vi "Reporte_Word.vi"() -> ()   [LabVIEW 2016]
uses:
  <vilib>/addons/_office/_exclsub.llb/font.ctl
  <vilib>/addons/_office/word.llb/Word Easy Table (num).vi
  <vilib>/Utility/NIReport.llb/Append Image to Report (path wrap).vi
  <vilib>/printing/ReportDocExtensions.llb/Append Front Panel Image to Report (path).vi
  <vilib>/printing/ReportDocExtensions.llb/Append VI Block Diagram to Report (path).vi
  <vilib>/Utility/NIReport.llb/NI_report.lvclass
  <vilib>/addons/_office/NI_ReportGenerationToolkit.lvlib
  <vilib>/Utility/NIReport.llb/NI_ReportGenerationCore.lvlib
panel:
  in  "VI":path
  in  "File Path Control":path
  out "Gauge":dbl(knob) scale=0.0..10.0
  in  "path or URL of image":path
  in  "Array":dbl[][](array[numeric])
  in  "String 2":string
  in  "String":string
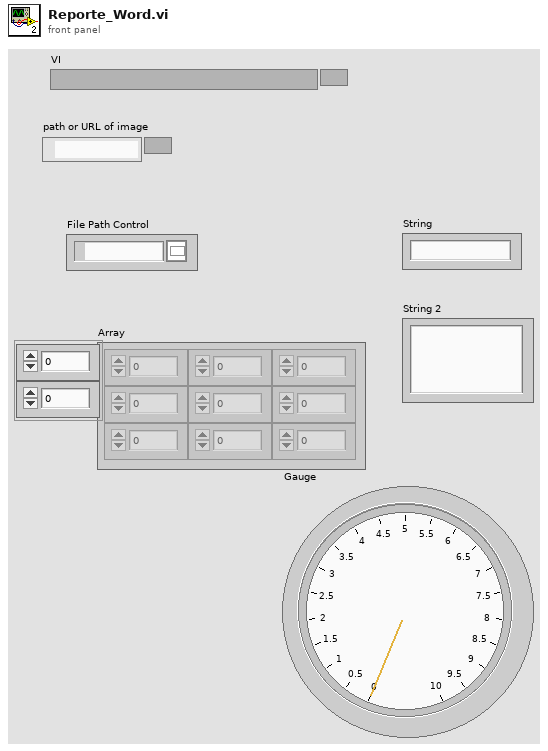
[diagram p1: front panel]
types:
  T1 = enum16{"xlColumnClustered", "xlColumnStacked", "xlColumnStacked100", "xl3DColumnClustered", "xl3DColumnStacked", "xl3DColumnStacked100", "xlBarClustered", "xlBarStacked", "xlBarStacked100", "xl3DBarClustered", "xl3DBarStacked", "xl3DBarStacked100", "xlLineStacked", "xlLineStacked100", "xlLineMarkers", "xlLineMarkersStacked", "xlLineMarkersStacked100", "xlPieOfPie", "xlPieExploded", "xl3DPieExploded", "xlBarOfPie", "xlXYScatterSmooth", "xlXYScatterSmoothNoMarkers", "xlXYScatterLines", "xlXYScatterLinesNoMarkers", "xlAreaStacked", "xlAreaStacked100", "xl3DAreaStacked", "xl3DAreaStacked100", "xlDoughnutExploded", "xlRadarMarkers", "xlRadarFilled", "xlSurface", "xlSurfaceWireframe", "xlSurfaceTopView", "xlSurfaceTopViewWireframe", "xlBubble", "xlBubble3DEffect", "xlStockHLC", "xlStockOHLC", "xlStockVHLC", "xlStockVOHLC", "xlCylinderColClustered", "xlCylinderColStacked", "xlCylinderColStacked100", "xlCylinderBarClustered", "xlCylinderBarStacked", "xlCylinderBarStacked100", "xlCylinderCol", "xlConeColClustered", "xlConeColStacked", "xlConeColStacked100", "xlConeBarClustered", "xlConeBarStacked", "xlConeBarStacked100", "xlConeCol", "xlPyramidColClustered", "xlPyramidColStacked", "xlPyramidColStacked100", "xlPyramidBarClustered", "xlPyramidBarStacked", "xlPyramidBarStacked100", "xlPyramidCol", "xl3DColumn", "xlLine", "xl3DLine", "xl3DPie", "xlPie", "xlXYScatter", "xl3DArea", "xlArea", "xlDoughnut", "xlRadar"}
  T2 = typedef "NI_ReportGenerationToolkit.lvlib/font.ctl" = cluster{"font name":string, "font size":dbl, "bold":u16, "italic":u16, "underline":u16, "strike through":u16, "font color":u32}
  T3 = enum16{"maximized", "minimized", "normal", "no change"}
  T4 = enum16{"Standard Report", "HTML", "Word", "Excel"}
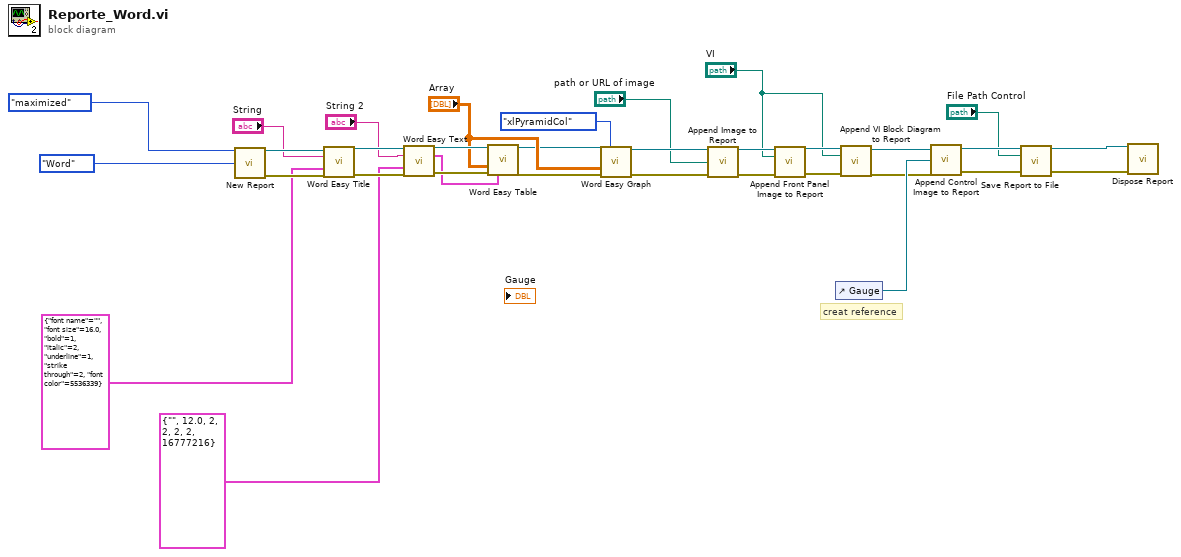
[diagram p0: block diagram]
diagram:
  # "creat reference"
  n1 = call <vilib>:"New Report.vi"("window state (normal)"=T3."maximized", "report type"=T4."Word") -> ("report out"=w31:refnum<class "NI_report.lvclass">, "error out"=w27:errorcluster)  [unwired: 12 in]
  n2 = call <vilib>:"Word Easy Title.vi"("report in"=w31, "title"="String", "font"=T2 {"font name"="", "font size"=16.0, "bold"=1, "italic"=2, "underline"=1, "strike through"=2, "font color"=5536339}, "error in (no error)"=w27) -> ("report out"=w29:refnum<class "NI_report.lvclass">, "error out"=w26:errorcluster)  [unwired: 9 in, 1 out]
  n3 = call <vilib>:"Word Easy Text.vi"("report in"=w29, "text"="String 2", "font"=T2 {"font name"="", "font size"=12.0, "bold"=2, "italic"=2, "underline"=2, "strike through"=2, "font color"=16777216}, "error in (no error)"=w26) -> ("report out"=w25:refnum<class "NI_report.lvclass">, "font out"=w21:T2, "error out"=w24:errorcluster)  [unwired: 9 in]
  n4 = call-poly <vilib>:"Word Easy Table.vi"("report in"=w25, "text data"="Array", "error in (no error)"=w24, "font"=w21) -> ("report out"=w18:refnum<class "NI_report.lvclass">, "error out"=w17:errorcluster)  [unwired: 9 in, 1 out]
  n5 = call <vilib>:"Word Easy Graph.vi"("report in"=w18, "graph type (col clustered)"=T1."xlPyramidCol", "data"="Array", "error in (no error)"=w17) -> ("report out"=w16:refnum<class "NI_report.lvclass">, "error out"=w15:errorcluster)  [unwired: 10 in]
  n6 = call-poly <vilib>:"Append Image to Report.vi"("report in"=w16, "path or URL of image"="path or URL of image", "error in (no error)"=w15) -> ("report out"=w5:refnum<class "NI_report.lvclass">, "error out"=w4:errorcluster)  [unwired: 9 in, 2 out]
  n7 = call-poly <vilib>:"Append Front Panel Image to Report.vi"("report in"=w5, "VI"="VI", "error in (no error)"=w4) -> ("report out"=w7:refnum<class "NI_report.lvclass">, "error out"=w6:errorcluster)  [unwired: 8 in, 3 out]
  n8 = control-ref of="Gauge"() -> (w13:refnum<vi>)
  n9 = call-poly <vilib>:"Append VI Block Diagram to Report.vi"("report in"=w7, "VI"="VI", "error in (no error)"=w6) -> ("report out"=w2:refnum<class "NI_report.lvclass">, "error out"=w1:errorcluster)  [unwired: 8 in, 3 out]
  n10 = call-dynamic "Append Control Image to Report.vi"("report in"=w2, "ctrl reference"=w13, "error in (no error)"=w1) -> ("report out"=w11:refnum<class "NI_report.lvclass">, "error out"=w12:errorcluster)  [unwired: 9 in, 2 out]
  n11 = call-dynamic "Save Report to File.vi"("report in"=w11, "report file path"="File Path Control", "error in (no error)"=w12) -> ("report out"=w9:refnum<class "NI_report.lvclass">, "error out"=w8:errorcluster)  [unwired: 11 in]
  n12 = call-dynamic "Dispose Report.vi"("report in"=w9, "error in (no error)"=w8) -> ()  [unwired: 13 in, 1 out]
